vi "Read Full Force Test Settings.vi"(8 "error in (no error)":errorcluster, 11 "Boot Loader in":refnum<class "Boot Loader.lvclass">) -> (0 "error out":errorcluster, 2 "Full Force Test Settings":T1 {"Tolerance %" format="%.4f"; "Process Time" format="%.4f"; "Sample Time" format="%.4f"; "Lateral Force 4" format="%.4f"; "Axial Force 4" format="%.4f"; "Lateral Force 3" format="%.4f"; "Axial Force 3" format="%.4f"; "Lateral Force 2" format="%.4f"; "Axial Force 2" format="%.4f"; "Axial Force 1" format="%.4f"; "Lateral Force 1" format="%.4f"}, 3 "Boot Loader out":refnum<class "Boot Loader.lvclass">)   [LabVIEW 2015, in "Boot Loader.lvclass"]
uses:
  Boot Loader.lvclass
  Typedefs/FullForceScanSettings.ctl
  Settings/Settings.lvclass
  Typedefs/FAMT Typedefs.lvlib
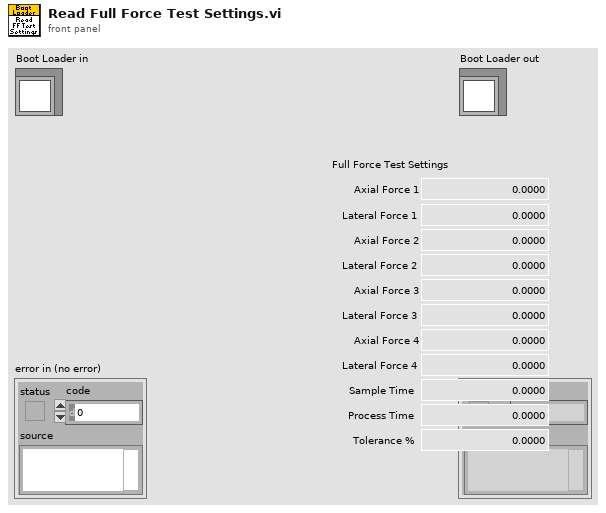
[diagram p1: front panel]
types:
  T1 = typedef "FAMT Typedefs.lvlib/FullForceScanSettings.ctl" = cluster{"Axial Force 1":dbl, "Lateral Force 1":dbl, "Axial Force 2":dbl, "Lateral Force 2":dbl, "Axial Force 3":dbl, "Lateral Force 3":dbl, "Axial Force 4":dbl, "Lateral Force 4":dbl, "Sample Time":dbl, "Process Time":dbl, "Tolerance %":dbl}
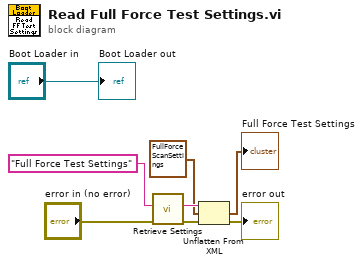
[diagram p0: block diagram]
diagram:
  n1 = call "Retrieve Settings.vi"("error in (no error)"="error in (no error)", "configName"="Full Force Test Settings") -> ("error out"=w4:errorcluster, "xmlConfig"=w7:string)  [unwired: 7 in, 1 out]
  n2 = Unflatten From XML(xml string=w7, type=T1 {"Axial Force 1"=0.0, "Lateral Force 1"=0.0, "Axial Force 2"=0.0, "Lateral Force 2"=0.0, "Axial Force 3"=0.0, "Lateral Force 3"=0.0, "Axial Force 4"=0.0, "Lateral Force 4"=0.0, "Sample Time"=0.0, "Process Time"=0.0, "Tolerance %"=0.0} ("Full Force Test Settings"), error in (no error)=w4) -> (value=→"Full Force Test Settings":T1, error out=→"error out":errorcluster)
  "Boot Loader out" <- "Boot Loader in"
